vi "Format Instance_System_StatusType_LVXML.vi"(8 "error in (no error)":errorcluster, 9 "Tag name":string, 10 "xmlData":T2, 11 "AWS_EC2 in":refnum<class "AWS_EC2.lvclass">) -> (0 "error out":errorcluster, 2 "InstaneStatusType":T3, 3 "AWS_EC2 out":refnum<class "AWS_EC2.lvclass">)   [LabVIEW 2014, in "AWS_EC2.lvlib" / "AWS_EC2.lvclass"]
uses:
  AWS_EC2.lvclass
  EC2 Datatypes/InstanceStatusType.ctl
  EC2 Datatypes/InstanceStatusDetailsSetType.ctl
  lv-xml-parser/r0/trunk/VI Source/EventType.ctl
  AWS_EC2.lvlib
  lv-xml-parser/r0/trunk/VI Source/LV XML Parser.lvlib
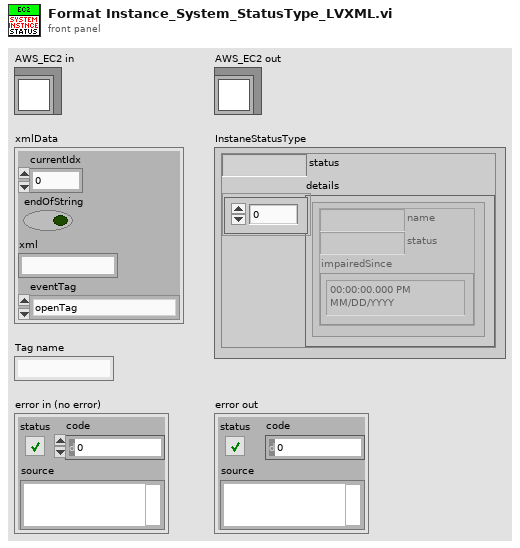
[diagram p1: front panel]
types:
  T1 = typedef "LV XML Parser.lvlib/EventType.ctl" = enum16{"openTag", "endOpenTag", "closeTag", "comment", "endComment", "endOfFile", "attribute", "startXml"}
  T2 = cluster{"currentIdx":i32, "endOfString":bool, "xml":string, "eventTag":T1}
  T3 = typedef "AWS_EC2.lvlib/InstanceStatusType.ctl" = cluster{"status":string, "details":T4[]}
  T4 = typedef "AWS_EC2.lvlib/InstanceStatusDetailsSetType.ctl" = cluster{"name":string, "status":string, "impairedSince":timestamp}
  T5 = cluster{"namespaceUri":string, "localName":string}
  T6 = cluster{"Attributes":cluster{"localName":string, "namespaceUri":string, "value":string}[], "localName":string, "namespaceUri":string, "valueXmlData":cluster{"currentIdx":i32, "endOfString":bool, "xml":string, "eventTag":T1}}[]
  T7 = cluster{"Attributes":cluster{"localName":string, "namespaceUri":string, "value":string}[], "localName":string, "namespaceUri":string, "valueXmlData":cluster{"currentIdx":i32, "endOfString":bool, "xml":string, "eventTag":T1}}
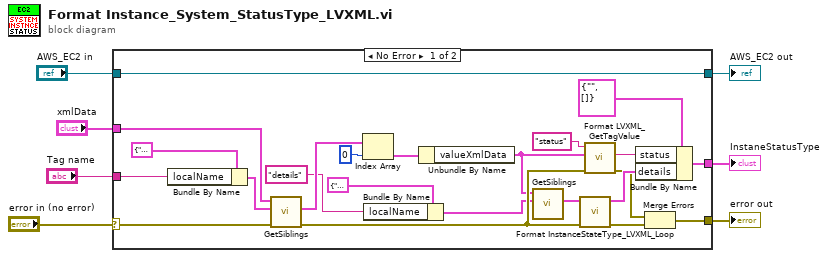
[diagram p0: block diagram]
diagram:
  n1 = case shown="No Error" "error in (no error)" {
    selector: "error in (no error)" -> [w25 w32]
    tunnel: "xmlData" -> [w28 _]
    tunnel: "AWS_EC2 in" -> [w27 w31]
    tunnel: [w27 w31] -> w4
    tunnel: "Tag name" -> [w26 _]
    tunnel: [w23 _] -> w6
    tunnel: [w16 w32] -> w7
    frame No Error {
      n2 = Bundle By Name(cluster=T5 {"namespaceUri"="", "localName"=""} ("limitToTag"), "localName"=w26) -> (w30:T5)
      n3 = call "GetSiblings.vi"("error in (no error)"=w25, "limitToTag"=w30, "xmlData"=w28) -> ("error out"=w13:errorcluster, "Siblings"=w17:T6)  [unwired: 7 in]
      n4 = Index Array(array=w17, index=0) -> (element=w22:T7)
      n5 = Bundle By Name(cluster=T5 {"namespaceUri"="", "localName"=""} ("limitToTag"), "localName"="details") -> (w11:T5)
      n6 = Unbundle By Name(w22) -> ("valueXmlData"=w12:T2)
      n7 = call "GetSiblings.vi"("limitToTag"=w11, "xmlData"=w12) -> ("Siblings"=w8:T6)  [unwired: 8 in, 1 out]
      n8 = call "Format InstanceStateType_LVXML_Loop.vi"("error in (no error)"=w13, "Siblings in"=w8) -> ("error out"=w14:errorcluster, "Array"=w18:T4[])  [unwired: 8 in]
      n9 = call "Format LVXML_GetTagValue.vi"("error in (no error)"=w13, "xmlDataIn"=w12, "Tag name"="status") -> ("error out"=w15:errorcluster, "Value"=w19:string)  [unwired: 6 in, 1 out]
      n10 = Bundle By Name(cluster=T3 {"status"="", "details"=[]} ("InstaneStatusType"), "status"=w19, "details"=w18) -> (w23:T3)
      n11 = Merge Errors(w15, w14) -> (w16:errorcluster)
    }
    frame Error {
    }
  }
  "error out" <- w7
  "InstaneStatusType" <- w6
  "AWS_EC2 out" <- w4
